vi "stim config control color update (sub-vi).vi"(8 "error in (no error)":errorcluster, 10 "odor-color map":T1, 11 "maifold config array refnum":refnum<vi>) -> (0 "error out":errorcluster, 3 "manifold config array refnum out":refnum<vi>)   [LabVIEW 2021]
uses:
  type-defs/odor channel to odor color map (type def).ctl
  type-defs/odor selection (type def).ctl
  type-defs/odor color (type def).ctl
  type-defs/odor color enum (type def).ctl
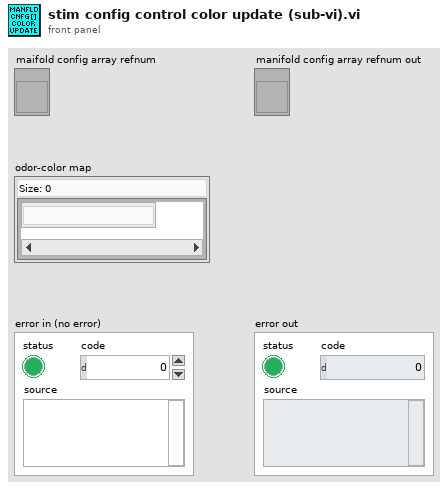
[diagram p1: front panel]
types:
  T1 = typedef "odor channel to odor color map (type def).ctl" = map{T2, T3}
  T2 = typedef "odor selection (type def).ctl" = enum16{"[none]", "odor 1", "odor 2", "odor 3", "odor 4", "odor 5", "odor 6", "odor 7", "odor 8", "odor 9", "odor 10"}
  T3 = typedef "odor color (type def).ctl" = u16
  T4 = typedef "odor color enum (type def).ctl" = enum16{"white", "blue", "red", "orange", "yellow", "green", "magenta", "brown", "black", "[none]"}
  T5 = typedef "stimulator configuration cluster (type def).ctl" = cluster{"position:":T6, "port connections:":T7[]}
  T6 = typedef "stimulator selection.ctl" = enum16{"left", "middle", "right"}
  T7 = typedef "single port single odor cluster.ctl" = cluster{"port number":T8, "connected odor":T2, "error":bool, "odor color":T3}
  T8 = typedef "port number (type def).ctl" = enum16{"port 1", "port 2", "port 3", "port 4", "port 5", "port 6", "port 7", "port 8"}
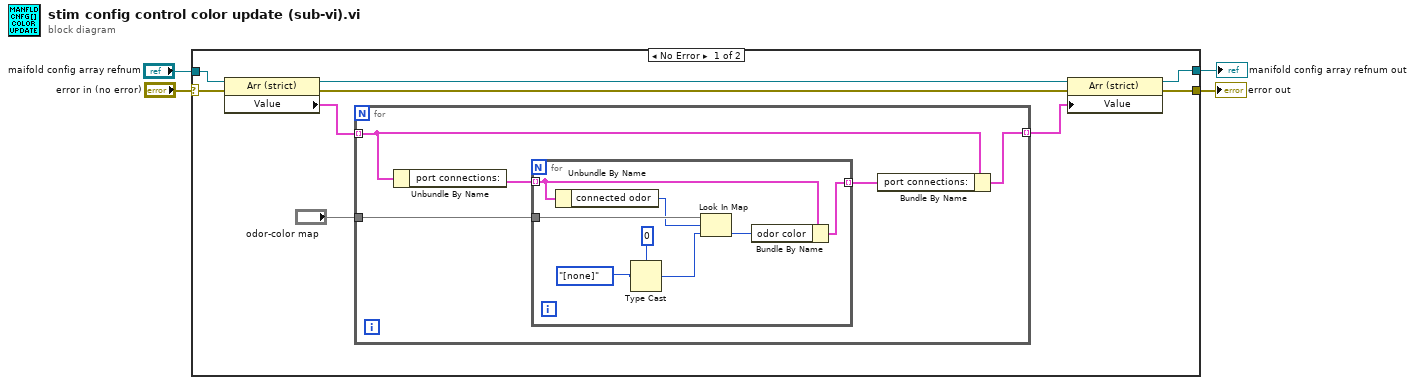
[diagram p0: block diagram]
diagram:
  n1 = case shown="No Error" "error in (no error)" {
    selector: "error in (no error)" -> [w11 w27]
    tunnel: [w13 w27] -> w4
    tunnel: [w6 w28] -> w2
    tunnel: "maifold config array refnum" -> [w5 w28]
    frame No Error {
      n2 = property class="Arr (strict)"(reference=w5, error in=w11) -> (reference out=w7:refnum<vi>, error out=w12:errorcluster, "Value"=w8:T5[])
      n3 = for {
        tunnel: w8 -> [w16] mode=indexing
        tunnel: "odor-color map" -> [w17]
        tunnel: [w14] -> w10 mode=indexing
        n4 = Unbundle By Name(w16) -> ("port connections:"=w18:T7[])
        n5 = for {
          tunnel: w18 -> [w24] mode=indexing
          tunnel: w17 -> [w26]
          tunnel: [w22] -> w15 mode=indexing
          n6 = Unbundle By Name(w24) -> ("connected odor"=w25:T2)
          n7 = Type Cast(type=T3 0 ("default value"), x=odor_color_enum_(type_def)."[none]" ("Enum")) -> (*(type *) &x=w19:T3)
          n8 = Look In Map(map=w26, key=w25, default value=w19) -> (value=w23:T3)  [unwired: 1 out]
          n9 = Bundle By Name(cluster=w24, "odor color"=w23) -> (w22:T7)
        }
        n10 = Bundle By Name(cluster=w16, "port connections:"=w15) -> (w14:T5)
      }
      n11 = property class="Arr (strict)"(reference=w7, error in=w12, "Value"=w10) -> (reference out=w6:refnum<vi>, error out=w13:errorcluster)
    }
    frame Error {
    }
  }
  "error out" <- w4
  "manifold config array refnum out" <- w2
